vi "IDS_rt_get_ResolutionSinCos.vi"(8 "error in (no error)":errorcluster, 11 "deviceHandle":i32) -> (0 "error out":errorcluster, 2 "resolution out":i32, 3 "deviceHandle out":i32)   [LabVIEW 2016]
doc: "int IDS_DLL IDS_rt_getResolutionSinCos(int32_t * resolution);"
panel:
  in  "resolution":i32
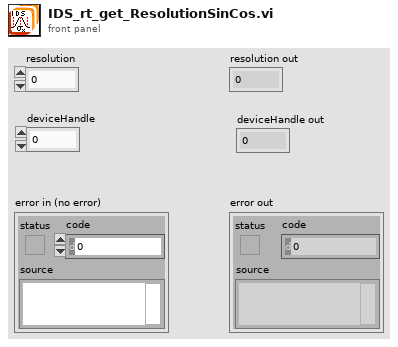
[diagram p1: front panel]
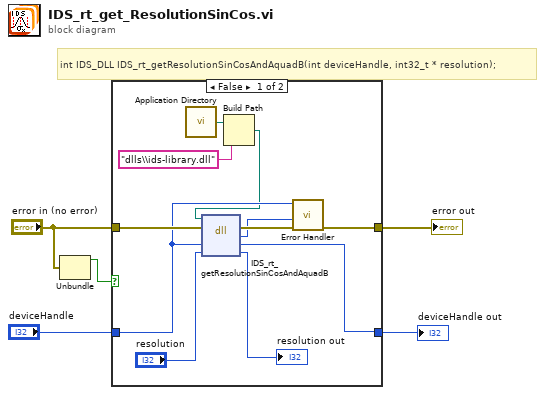
[diagram p0: block diagram]
diagram:
  # "int IDS_DLL IDS_rt_getResolutionSinCosAndAquadB(int deviceHandle, int32_t * resolution);"
  n1 = Unbundle("error in (no error)") -> ("status"=w1:bool)  [unwired: 2 out]
  n2 = case shown="False" w1 {
    tunnel: "error in (no error)" -> [w15 w18]
    tunnel: [w16 w18] -> w5
    tunnel: "deviceHandle" -> [w9 w17]
    tunnel: [w11 w17] -> w3
    frame False {
      n3 = call <vilib>:"Application Directory.vi"() -> ("Application Directory"=w8:path)
      n4 = Build Path(base path=w8, name or relative path="dlls\\ids-library.dll" ("ipAddress")) -> (appended path=w6:path)
      n5 = dll-call lib="C:/Users/matheus/Desktop/LabVIEW_Draft_V1.6.0/dlls/ids-library.dll" fn="IDS_rt_getResolutionSinCosAndAquadB"(path in=w6, error in=w15, "deviceHandle"=w9, "resolution"="resolution") -> (error out=w14:errorcluster, "return type"=w10:i32, "deviceHandle"=w11:i32, "resolution"=→"resolution out":i32)  [unwired: 1 in, 1 out]
      n6 = call "Error Handler.vi"("error in (no error)"=w14, "error code"=w10, "deviceHandle"=w9) -> ("error out"=w16:errorcluster)  [unwired: 7 in, 1 out]
    }
    frame True {
    }
  }
  "error out" <- w5
  "deviceHandle out" <- w3
